vi "Main.vi"() -> ()   [LabVIEW 2015, in "ModbusOverMOXA.lvlib"]
doc: "This template is based from the Queued Message Handler design pattern and the Queued Message Handler Project Template that ships with LabVIEW 2014.\n\nThe main difference is that the Queue is private to this module and communication between modules is done via Broadcast and Requests events.\n\nRequests events are wrapped via public API methods and are handled in the Event handler loop in this VI.\nAny module can register for Broadcast events sent by this module.\n\nThe Event Handling Loop generates messages based on user interface actions.\n\nThe Message Handling Loop processes messages generated by the Event Handling Loop, or by other messages. The messages are string values, so new messages can be added easily to the Message Cases case structure in the Message Handling Loop. Each message cluster can also provide an optional value for Message Data, which is a variant that can be converted to whatever message-specific data is required.\n_____\nBased on Delacor QMH Project Template 3.1.0.34."
uses:
  ModbusOverMOXA.lvlib
  <vilib>/Delacor/Delacor QMH/Libraries/Cloneable Module Admin_class/Delacor_lib_QMH_Cloneable Module Admin.lvclass
  libs/ModBUS.lvlibp/RTU/RTU.lvclass
  Module Data--cluster.ctl
  libs/ModBUS.lvlibp/Base/Modbus.lvclass
  Command.ctl
  <vilib>/Delacor/Delacor QMH/Libraries/Cloneable Module Admin_class/Delacor_lib_QMH_Cloneable Module Admin.lvclass/Delacor_lib_QMH_Cloneable Module Admin.ctl
  Stop Argument--cluster.ctl
  <vilib>/Delacor/Delacor QMH/Libraries/Module Admin_class/Delacor_lib_QMH_Module Admin.lvclass/Delacor_lib_QMH_Module Admin.ctl
  Configure Argument--cluster.ctl
  SetRemote Argument--cluster.ctl
  GetStatus Argument--cluster.ctl
  Drive Argument--cluster.ctl
  ReadRegister Argument--cluster.ctl
  WriteRegister Argument--cluster.ctl
  <vilib>/Utility/miscctls.llb/LVPointTypeDef.ctl
  engage Argument--cluster.ctl
  <vilib>/Delacor/Delacor QMH/Libraries/Cloneable Module Admin_class/Delacor_lib_QMH_Get Module ID.vi
  <vilib>/Delacor/Delacor QMH/Libraries/Module Admin_class/Delacor_lib_QMH_Get External Launch.vi
  <vilib>/Delacor/Delacor QMH/Libraries/Message Queue_class/Delacor_lib_QMH_Enqueue Message (Single).vi
  <vilib>/Utility/error.llb/Error Cluster From Error Code.vi
  <vilib>/ErrorRing/Error Ring.xnode
  <vilib>/Delacor/Delacor QMH/Libraries/Message Queue_class/Delacor_lib_QMH_Message Queue.lvclass
  Clone Registration/Clone Registration.lvlib
  libs/Serializer.lvlibp
  libs/MQTT.lvlibp
panel:
  in  "Simulate MHL Error":bool
  in  "Simulate EHL Error":bool
  out "error out":errorcluster
  in  "Module Admin":refnum<class "Delacor_lib_QMH_Cloneable Module Admin.lvclass">
  out "Status":string
  # "Other QMH Modules communicate with this Module via its Public API (wrappers for its Request Events).\n\nThis Module communicates with other Modules via its Broadcast Events.\nAny module that wants to get these messages, just registers for this module's Broadcast events."
  # "This template is for the Delacor Modified Queued Message Handler design pattern.\n\nSee the block diagram for more information on how to use this template."
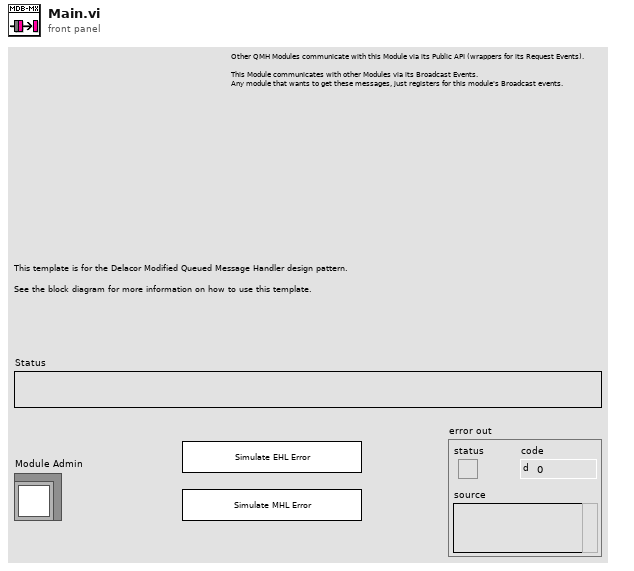
[diagram p1: front panel]
types:
  T1 = typedef "ModbusOverMOXA.lvlib/Request Events--cluster.ctl" = cluster{"Stop Module":refnum<user-event>, "Show Panel":refnum<user-event>, "Hide Panel":refnum<user-event>, "Show Diagram":refnum<user-event>, "Get Module Execution Status":refnum<user-event>, "Configure":refnum<user-event>, "SetRemote":refnum<user-event>, "GetStatus":refnum<user-event>, "engage":refnum<user-event>, "Drive":refnum<user-event>, "ReadRegister":refnum<user-event>, "WriteRegister":refnum<user-event>}
  T2 = typedef "Serializer.lvlibp/Broadcast Events--cluster.ctl" = cluster{"Module Did Init":refnum<user-event>, "Status Updated":refnum<user-event>, "Error Reported":refnum<user-event>, "Module Did Stop":refnum<user-event>, "Update Module Execution Status":refnum<user-event>, "Received":refnum<user-event>}
  T3 = typedef "MQTT.lvlibp/Broadcast Events--cluster.ctl" = cluster{"Module Did Init":refnum<user-event>, "Status Updated":refnum<user-event>, "Error Reported":refnum<user-event>, "Module Did Stop":refnum<user-event>, "Update Module Execution Status":refnum<user-event>, "Message":refnum<user-event>}
  T4 = typedef "ModbusOverMOXA.lvlib/Module Data--cluster.ctl" = cluster{"Status":string, "ModBUS":refnum<class "Modbus.lvclass">, "BitewiseCommand":cluster{"Register":dbl, "Command":string}, "Broadcasts":variant, "Subscriptions":variant, "commands queue":refnum<queue>, "Processing":bool, "processed command":T5, "StatusUpdate":timestamp}
  T5 = typedef "Command.ctl" = cluster{"Command":string, "ByteArray":u8[], "Finished":bool, "Time Stamp":timestamp}
  T6 = typedef "ModbusOverMOXA.lvlib/Stop Argument--cluster.ctl" = cluster{"Origin":string, "Module ID":i32, "Exit via Stop Module Req?":bool, "Wait for Module to stop?":bool}
  T7 = typedef "ModbusOverMOXA.lvlib/Configure Argument--cluster.ctl" = cluster{"Module ID":i32, "Jsonconfig":string}
  T8 = typedef "ModbusOverMOXA.lvlib/SetRemote Argument--cluster.ctl" = cluster{"Module ID":i32, "Remote?":bool}
  T9 = typedef "ModbusOverMOXA.lvlib/GetStatus Argument--cluster.ctl" = cluster{"Module ID":i32, "Boolean":bool}
  T10 = typedef "ModbusOverMOXA.lvlib/Drive Argument--cluster.ctl" = cluster{"Module ID":i32, "Hz":dbl}
  T11 = typedef "ModbusOverMOXA.lvlib/ReadRegister Argument--cluster.ctl" = cluster{"Module ID":i32, "Register":u16, "Length":u16}
  T12 = typedef "ModbusOverMOXA.lvlib/WriteRegister Argument--cluster.ctl" = cluster{"Module ID":i32, "Register":u16, "Data":u16}
  T13 = typedef "LVPointTypeDef.ctl" = cluster{"Horizontal":i16, "Vertical":i16}
  T14 = enum32{"Invalid", "Standard", "Closed", "Hidden", "Minimized", "Maximized"}
  T15 = enum32{"invalid lock state", "Not Locked", "Locked (No Password)", "Password-protected"}
  T16 = typedef "ModbusOverMOXA.lvlib/engage Argument--cluster.ctl" = cluster{"Module ID":i32, "Engage":bool}
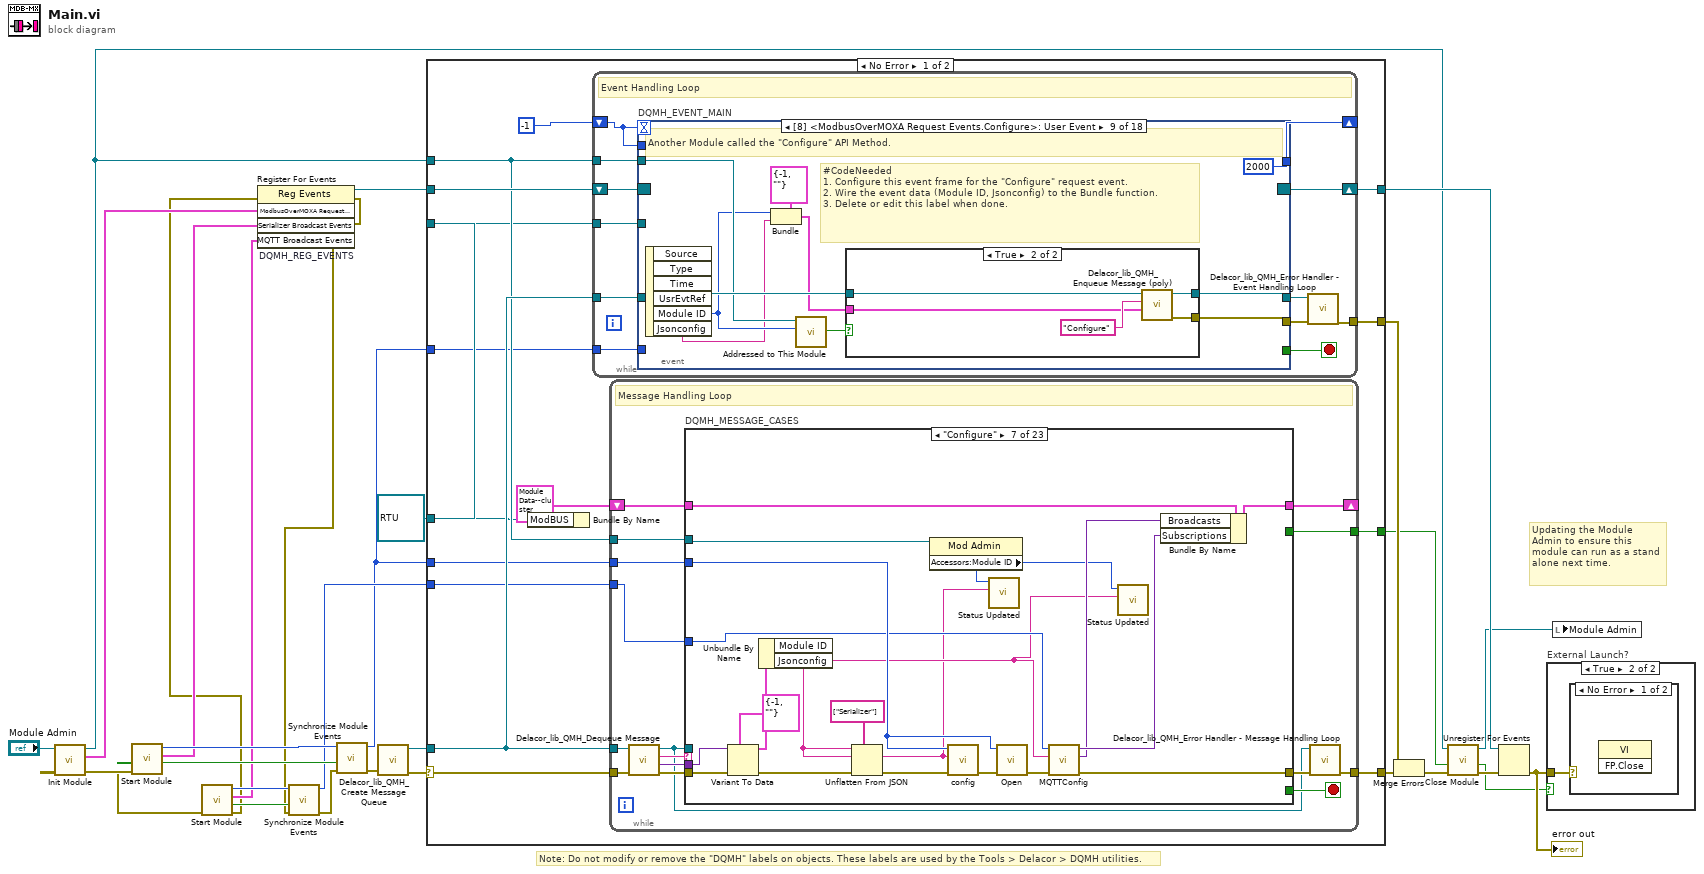
[diagram p0: block diagram]
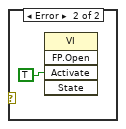
[diagram p3: hidden frame]
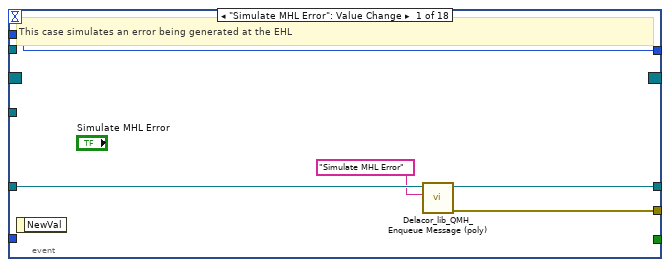
[diagram p4: hidden frame]
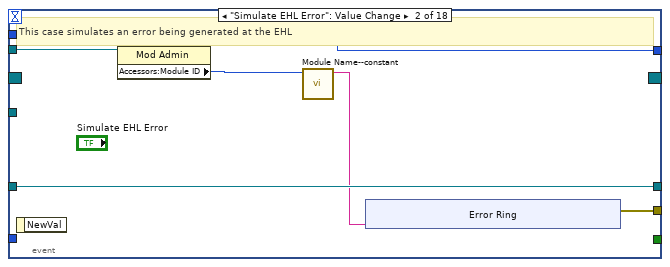
[diagram p5: hidden frame]
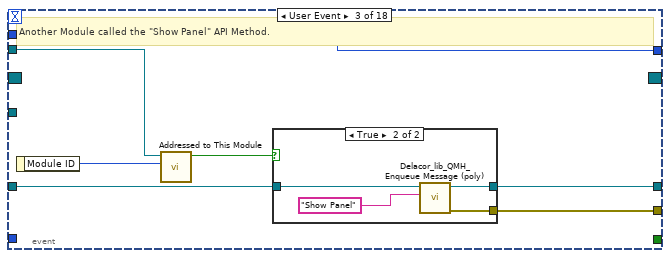
[diagram p6: hidden frame]
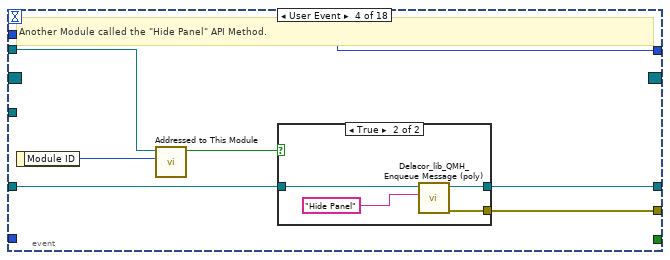
[diagram p8: hidden frame]
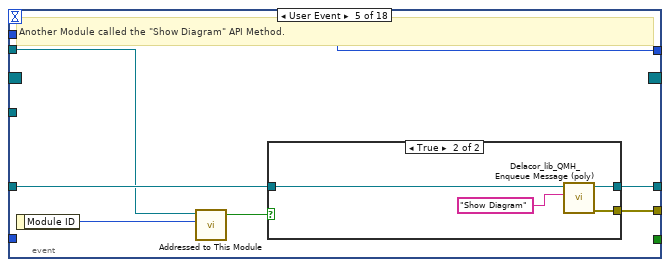
[diagram p10: hidden frame]
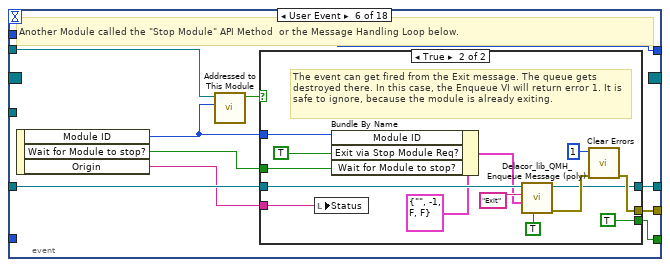
[diagram p12: hidden frame]
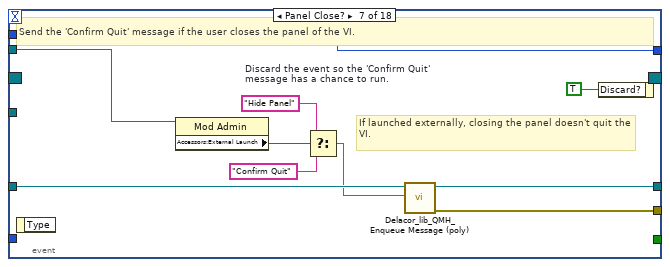
[diagram p14: hidden frame]
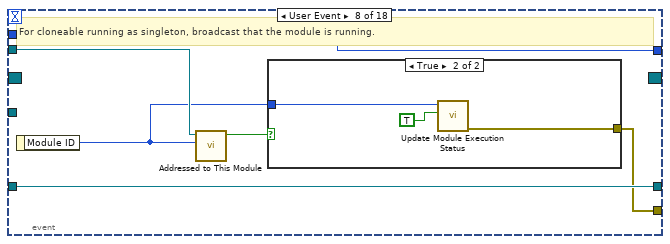
[diagram p15: hidden frame]
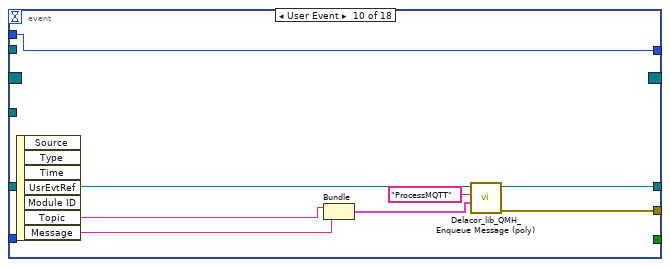
[diagram p18: hidden frame]
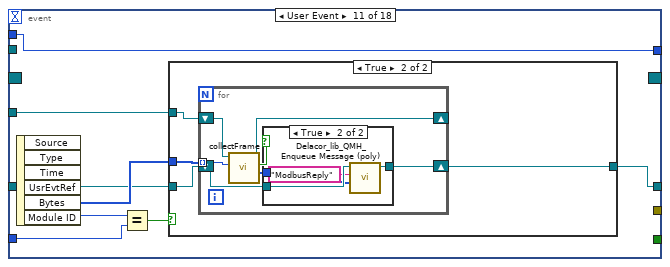
[diagram p19: hidden frame]
diagram:
  w1 = refnum<class "RTU.lvclass"> refnum ("ModBUS.lvlibp:RTU.lvclass")
  # "Note: Do not modify or remove the \"DQMH\" labels on objects. These labels are used by the Tools > Delacor > DQMH utilities."
  # "Updating the Module Admin to ensure this module can run as a stand alone next time."
  n1 = call "Init Module.vi"("Cloneable Module Admin in"="Module Admin") -> ("error out"=w11:errorcluster, "ModbusOverMOXA Request Events"=w25:T1, "Cloneable Module Admin out"=w21:refnum<class "Delacor_lib_QMH_Cloneable Module Admin.lvclass">)  [unwired: 8 in]
  n2 = call "Start Module.vi"("error in (no error)"=w11) -> ("error out"=w4:errorcluster, "Wait for Event Sync?"=w13:bool, "Serializer Broadcast Events"=w12:T2, "Module ID"=w14:i32)  [unwired: 7 in]
  n3 = call "Start Module.vi"("error in (no error)"=w4) -> ("error out"=w3:errorcluster, "Wait for Event Sync?"=w9:bool, "MQTT Broadcast Events"=w8:T3, "Module ID"=w10:i32)  [unwired: 7 in]
  n4 = register-events "DQMH_REG_EVENTS"(error in=w3, w25, w12, w8) -> (reference out=w26:refnum<event-registration>, error out=w6:errorcluster)  [unwired: 1 in]
  n5 = call "Synchronize Module Events.vi"("error in (no error)"=w6, "Wait for Event Sync?"=w9, "Module ID"=w10) -> ("error out"=w5:errorcluster, "Module ID (dup)"=w7:i32)  [unwired: 7 in]
  n6 = call "Synchronize Module Events.vi"("error in (no error)"=w5, "Wait for Event Sync?"=w13, "Module ID"=w14) -> ("error out"=w15:errorcluster, "Module ID (dup)"=w2:i32)  [unwired: 7 in]
  n7 = call <vilib>:"Delacor_lib_QMH_Create Message Queue.vi"("error in (no error)"=w15) -> ("error out"=w16:errorcluster, "Message Queue out"=w24:refnum<class "Delacor_lib_QMH_Message Queue.lvclass">)  [unwired: 9 in]
  n8 = case shown="No Error" w16 {
    selector: w16 -> [w40 w789]
    tunnel: [w46 w789] -> w28
    tunnel: [w45 w790] -> w27
    tunnel: w26 -> [w43 w790]
    tunnel: w24 -> [w42 _]
    tunnel: [w41 _] -> w29
    tunnel: w21 -> [w39 w785]
    tunnel: [w38 _] -> w19
    tunnel: w2 -> [w37 _]
    tunnel: w7 -> [w36 _]
    tunnel: w2 -> [w35 _]
    tunnel: w1 -> [w33 _]
    tunnel: w1 -> [w32 _]
    frame No Error {
      n9 = Bundle By Name(cluster=T4 {"Status"="", "ModBUS"=refnum, "BitewiseCommand"={"Register"=0.0, "Command"=""}, "Broadcasts"=variant, "Subscriptions"=variant, "commands queue"=refnum, "Processing"=FALSE, "processed command"={"Command"="", "ByteArray"=[], "Finished"=FALSE, "Time Stamp"=timestamp(0 s since 1904-01-01)}, "StatusUpdate"=timestamp(0 s since 1904-01-01)} ("Data Cluster"), "ModBUS"=w33) -> (w34:T4)
      n10 = while {
        tunnel: w42 -> [w58]
        shift-right: [w56] -> w45
        shift-left: w43 -> [w57]
        tunnel: [w52] -> w41
        tunnel: w39 -> [w51]
        tunnel: w35 -> [w50]
        tunnel: w32 -> [w49]
        shift-right: [w48] -> _
        shift-left: -1 -> [w47]
        stop <- w54 stop-if-true
        # "Event Handling Loop"
        n11 = event "DQMH_EVENT_MAIN" shown="[8] <ModbusOverMOXA Request Events.Configure>: User Event" {
          selector: w57 -> [_ _ _ _ _ _ _ _ _ _ _ _ _ _ _ _ _ _]
          dyn-events: [_ _ _ _ _ _ _ _ _ _ _ _ _ _ _ _ _ _] -> w56
          timeout: w47 -> [_ _ _ _ _ _ _ _ _ _ _ _ _ _ _ _ _ _]
          tunnel: [_ _ _ _ _ w117 _ _ _ _ _ _ _ _ _ _ _ _] -> w54
          tunnel: w58 -> [w63 w69 w83 w95 w107 w120 w146 w151 w166 w179 w183 w215 w231 w242 w251 w267 w284 w301]
          tunnel: [w61 w68 w81 w93 w103 w122 w145 w150 w160 w177 _ w209 w225 w240 w246 w261 w278 w295] -> w55
          tunnel: [w62 w69 w82 w94 w106 w121 w144 w151 w165 w178 w182 w214 w230 w241 w250 w266 w283 w300] -> w53
          tunnel: w51 -> [_ w67 w78 w90 w104 w119 w140 w152 w163 _ _ w212 w228 _ w248 w264 w281 w298]
          tunnel: w50 -> [_ _ _ _ _ _ _ _ _ _ w187 _ _ _ _ _ _ _]
          tunnel: w49 -> [_ _ _ _ _ _ _ _ _ _ w184 _ _ _ _ _ _ _]
          tunnel: [w59 w64 w77 w89 w101 w113 w138 w148 2000 w180 w181 w206 w222 w238 w243 w258 w274 w291] -> w48
          tunnel: w47 -> [w59 w64 w77 w89 w101 w113 w138 w148 _ w180 w181 w206 w222 w238 w243 w258 w274 w291]
          event "Simulate MHL Error": Value Change {
            # "This case simulates an error being generated at the EHL"
            n12 = event-data() -> ()  [unwired: 1 in, 1 out]
            n13 = call-poly <vilib>:"Delacor_lib_QMH_Enqueue Message (poly).vi"("Message"="Simulate MHL Error", "Message Queue in"=w63) -> ("error out"=w61:errorcluster, "Message Queue out"=w62:refnum<class "Delacor_lib_QMH_Message Queue.lvclass">)  [unwired: 8 in]
          }
          event "Simulate EHL Error": Value Change {
            # "This case simulates an error being generated at the EHL"
            n14 = event-data() -> ()  [unwired: 1 in, 1 out]
            n15 = property class="Mod Admin"(reference=w67) -> ("Accessors:Module ID"=w66:i32)  [unwired: 1 in, 2 out]
            n16 = call "Module Name--constant.vi"("Module ID"=w66) -> ("Module Name"=w65:string)  [unwired: 10 in]
            n17 = xnode "Error Ring"("parameter 0"=w65) -> ("error out"=w68:errorcluster)
          }
          event User Event {
            # "Another Module called the \"Show Panel\" API Method."
            n18 = event-data() -> ("Module ID"=w80:i32)  [unwired: 1 in]
            n19 = call "Addressed to This Module.vi"("Module ID from Argument"=w80, "Module Admin"=w78) -> ("Addressed to this instance?"=w79:bool)  [unwired: 8 in, 1 out]
            n20 = case shown="True" w79 {
              tunnel: w83 -> [w84 w88]
              tunnel: [w84 w87] -> w82
              tunnel: [_ w86] -> w81
              frame False {
              }
              frame True {
                n21 = call-poly <vilib>:"Delacor_lib_QMH_Enqueue Message (poly).vi"("Message"="Show Panel", "Message Queue in"=w88) -> ("error out"=w86:errorcluster, "Message Queue out"=w87:refnum<class "Delacor_lib_QMH_Message Queue.lvclass">)  [unwired: 8 in]
              }
            }
          }
          event User Event {
            # "Another Module called the \"Hide Panel\" API Method."
            n22 = event-data() -> ("Module ID"=w92:i32)  [unwired: 1 in]
            n23 = call "Addressed to This Module.vi"("Module ID from Argument"=w92, "Module Admin"=w90) -> ("Addressed to this instance?"=w91:bool)  [unwired: 8 in, 1 out]
            n24 = case shown="True" w91 {
              tunnel: w95 -> [w96 w100]
              tunnel: [w96 w99] -> w94
              tunnel: [_ w98] -> w93
              frame False {
              }
              frame True {
                n25 = call-poly <vilib>:"Delacor_lib_QMH_Enqueue Message (poly).vi"("Message"="Hide Panel", "Message Queue in"=w100) -> ("error out"=w98:errorcluster, "Message Queue out"=w99:refnum<class "Delacor_lib_QMH_Message Queue.lvclass">)  [unwired: 8 in]
              }
            }
          }
          event User Event {
            # "Another Module called the \"Show Diagram\" API Method."
            n26 = event-data() -> ("Module ID"=w102:i32)  [unwired: 1 in]
            n27 = call "Addressed to This Module.vi"("Module ID from Argument"=w102, "Module Admin"=w104) -> ("Addressed to this instance?"=w105:bool)  [unwired: 8 in, 1 out]
            n28 = case shown="True" w105 {
              tunnel: w107 -> [w108 w112]
              tunnel: [w108 w111] -> w106
              tunnel: [_ w109] -> w103
              frame False {
              }
              frame True {
                n29 = call-poly <vilib>:"Delacor_lib_QMH_Enqueue Message (poly).vi"("Message"="Show Diagram", "Message Queue in"=w112) -> ("error out"=w109:errorcluster, "Message Queue out"=w111:refnum<class "Delacor_lib_QMH_Message Queue.lvclass">)  [unwired: 8 in]
              }
            }
          }
          event User Event {
            # "Another Module called the \"Stop Module\" API Method  or the Message Handling Loop below."
            n30 = event-data() -> ("Module ID"=w115:i32, "Wait for Module to stop?"=w116:bool, "Origin"=w114:string)  [unwired: 1 in]
            n31 = call "Addressed to This Module.vi"("Module ID from Argument"=w115, "Module Admin"=w119) -> ("Addressed to this instance?"=w118:bool)  [unwired: 8 in, 1 out]
            n32 = case shown="True" w118 {
              tunnel: [_ w133] -> w122
              tunnel: [w123 w132] -> w121
              tunnel: w120 -> [w123 w131]
              tunnel: [_ TRUE] -> w117
              tunnel: w116 -> [_ w126]
              tunnel: w115 -> [_ w128]
              tunnel: w114 -> [_ w124]
              frame False {
              }
              frame True {
                # "The event can get fired from the Exit message. The queue gets destroyed there. In this case, the Enqueue VI will return error 1. It is safe to ignore, because the module is already exiting."
                n33 = local write "Status"(w124) -> ()
                n34 = Bundle By Name(cluster=T6 {"Origin"="", "Module ID"=-1, "Exit via Stop Module Req?"=FALSE, "Wait for Module to stop?"=FALSE} ("Stop Argument"), "Module ID"=w128, "Exit via Stop Module Req?"=TRUE, "Wait for Module to stop?"=w126) -> (w125:T6)
                n35 = call-poly <vilib>:"Delacor_lib_QMH_Enqueue Message (poly).vi"("Priority Message? (F)"=TRUE, "Message Data"=w125, "Message"="Exit", "Message Queue in"=w131) -> ("error out"=w136:errorcluster, "Message Queue out"=w132:refnum<class "Delacor_lib_QMH_Message Queue.lvclass">)  [unwired: 6 in]
                n36 = call <vilib>:"Clear Errors.vi"("error in (no error)"=w136, "specific error code to clear (0: all)"=1) -> ("error out"=w133:errorcluster)  [unwired: 4 in, 1 out]
              }
            }
          }
          event Panel Close? {
            w147 = TRUE  # Discard the event so the 'Confirm Quit' message has a chance to run.
            # "If launched externally, closing the panel doesn't quit the VI."
            # "Send the 'Confirm Quit' message if the user closes the panel of the VI."
            n37 = event-data() -> ()  [unwired: 1 in, 1 out]
            n38 = property class="Mod Admin"(reference=w140) -> ("Accessors:External Launch"=w139:bool)  [unwired: 1 in, 2 out]
            n39 = Select(t="Hide Panel" ("Message"), s=w139, f="Confirm Quit" ("Message")) -> (s? t:f=w141:string)
            n40 = call-poly <vilib>:"Delacor_lib_QMH_Enqueue Message (poly).vi"("Message"=w141, "Message Queue in"=w146) -> ("error out"=w145:errorcluster, "Message Queue out"=w144:refnum<class "Delacor_lib_QMH_Message Queue.lvclass">)  [unwired: 8 in]
            n41 = event-data("Discard?"=w147) -> ()  [unwired: 1 in, 1 out]
          }
          event User Event {
            # "For cloneable running as singleton, broadcast that the module is running."
            n42 = event-data() -> ("Module ID"=w149:i32)  [unwired: 1 in]
            n43 = call "Addressed to This Module.vi"("Module ID from Argument"=w149, "Module Admin"=w152) -> ("Addressed to this instance?"=w153:bool)  [unwired: 8 in, 1 out]
            n44 = case shown="True" w153 {
              tunnel: [_ w156] -> w150
              tunnel: w149 -> [_ w155]
              frame False {
              }
              frame True {
                n45 = call "Update Module Execution Status.vi"("Running?"=TRUE, "Module ID"=w155) -> ("error out"=w156:errorcluster)  [unwired: 9 in]
              }
            }
          }
          event User Event {
            # "#CodeNeeded\n1. Configure this event frame for the \"Configure\" request event.\n2. Wire the event data (Module ID, Jsonconfig) to the Bundle function.\n3. Delete or edit this label when done."
            # "Another Module called the \"Configure\" API Method."
            n46 = event-data() -> ("Module ID"=w159:i32, "Jsonconfig"=w158:string)  [unwired: 1 in, 4 out]
            n47 = Bundle(cluster=T7 {"Module ID"=-1, "Jsonconfig"=""} ("Configure Argument"), "Module ID"=w159, "Jsonconfig"=w158) -> (w161:T7)
            n48 = call "Addressed to This Module.vi"("Module ID from Argument"=w159, "Module Admin"=w163) -> ("Addressed to this instance?"=w164:bool)  [unwired: 8 in, 1 out]
            n49 = case shown="True" w164 {
              tunnel: w166 -> [w167 w172]
              tunnel: [w167 w171] -> w165
              tunnel: w161 -> [_ w169]
              tunnel: [_ w168] -> w160
              frame False {
              }
              frame True {
                n50 = call-poly <vilib>:"Delacor_lib_QMH_Enqueue Message (poly).vi"("Message Data"=w169, "Message"="Configure", "Message Queue in"=w172) -> ("error out"=w168:errorcluster, "Message Queue out"=w171:refnum<class "Delacor_lib_QMH_Message Queue.lvclass">)  [unwired: 7 in]
              }
            }
          }
          event User Event {
            n51 = event-data() -> ("Topic"=w175:string, "Message"=w174:string)  [unwired: 1 in, 5 out]
            n52 = Bundle("Topic"=w175, "Message"=w174) -> (w173:cluster{"Topic":string, "Message":string})  [unwired: 1 in]
            n53 = call-poly <vilib>:"Delacor_lib_QMH_Enqueue Message (poly).vi"("Message Data"=w173, "Message"="ProcessMQTT", "Message Queue in"=w179) -> ("error out"=w177:errorcluster, "Message Queue out"=w178:refnum<class "Delacor_lib_QMH_Message Queue.lvclass">)  [unwired: 7 in]
          }
          event User Event {
            n54 = event-data() -> ("Bytes"=w185:u8[], "Module ID"=w188:i32)  [unwired: 1 in, 4 out]
            n55 = Equal?(x=w188, y=w187) -> (x = y?=w186:bool)
            n56 = case shown="True" w186 {
              tunnel: w185 -> [_ w193]
              tunnel: w184 -> [_ w192]
              tunnel: w183 -> [w189 w191]
              tunnel: [w189 w190] -> w182
              frame False {
              }
              frame True {
                n57 = for {
                  tunnel: w193 -> [w199] mode=indexing
                  shift-right: [w197] -> _
                  shift-left: w192 -> [w200]
                  shift-right: [w194] -> w190
                  shift-left: w191 -> [w195]
                  n58 = call-dynamic "collectFrame.vi"("byte"=w199, "RTU in"=w200) -> ("Data"=w196:i16[], "Finished"=w198:bool, "RTU out"=w197:refnum<class "RTU.lvclass">)  [unwired: 5 in, 2 out]
                  n59 = case shown="True" w198 {
                    tunnel: w196 -> [_ w204]
                    tunnel: w195 -> [w201 w205]
                    tunnel: [w201 w202] -> w194
                    frame False {
                    }
                    frame True {
                      n60 = call-poly <vilib>:"Delacor_lib_QMH_Enqueue Message (poly).vi"("Message Data"=w204, "Message"="ModbusReply", "Message Queue in"=w205) -> ("Message Queue out"=w202:refnum<class "Delacor_lib_QMH_Message Queue.lvclass">)  [unwired: 7 in, 1 out]
                    }
                  }
                }
              }
            }
          }
          event User Event {
            # "#CodeNeeded\n1. Configure this event frame for the \"SetRemote\" request event.\n2. Wire the event data (Module ID, Remote?) to the Bundle function.\n3. Delete or edit this label when done."
            # "Another Module called the \"SetRemote\" API Method."
            n61 = event-data() -> ("Module ID"=w208:i32, "Remote?"=w207:bool)  [unwired: 1 in, 4 out]
            n62 = Bundle(cluster=T8 {"Module ID"=-1, "Remote?"=FALSE} ("SetRemote Argument"), "Module ID"=w208, "Remote?"=w207) -> (w210:T8)
            n63 = call "Addressed to This Module.vi"("Module ID from Argument"=w208, "Module Admin"=w212) -> ("Addressed to this instance?"=w213:bool)  [unwired: 8 in, 1 out]
            n64 = case shown="True" w213 {
              tunnel: w215 -> [w216 w221]
              tunnel: [w216 w220] -> w214
              tunnel: w210 -> [_ w218]
              tunnel: [_ w217] -> w209
              frame False {
              }
              frame True {
                n65 = call-poly <vilib>:"Delacor_lib_QMH_Enqueue Message (poly).vi"("Message Data"=w218, "Message"="SetRemote", "Message Queue in"=w221) -> ("error out"=w217:errorcluster, "Message Queue out"=w220:refnum<class "Delacor_lib_QMH_Message Queue.lvclass">)  [unwired: 7 in]
              }
            }
          }
          event User Event {
            # "#CodeNeeded\n1. Configure this event frame for the \"GetStatus\" request event.\n2. Wire the event data (Module ID, Boolean) to the Bundle function.\n3. Delete or edit this label when done."
            # "Another Module called the \"GetStatus\" API Method."
            n66 = event-data() -> ("Module ID"=w223:i32, "Boolean"=w224:bool)  [unwired: 1 in, 4 out]
            n67 = Bundle(cluster=T9 {"Module ID"=-1, "Boolean"=FALSE} ("GetStatus Argument"), "Module ID"=w223, "Boolean"=w224) -> (w226:T9)
            n68 = call "Addressed to This Module.vi"("Module ID from Argument"=w223, "Module Admin"=w228) -> ("Addressed to this instance?"=w229:bool)  [unwired: 8 in, 1 out]
            n69 = case shown="True" w229 {
              tunnel: w231 -> [w232 w237]
              tunnel: [w232 w236] -> w230
              tunnel: w226 -> [_ w234]
              tunnel: [_ w233] -> w225
              frame False {
              }
              frame True {
                n70 = call-poly <vilib>:"Delacor_lib_QMH_Enqueue Message (poly).vi"("Message Data"=w234, "Message"="GetStatus", "Message Queue in"=w237) -> ("error out"=w233:errorcluster, "Message Queue out"=w236:refnum<class "Delacor_lib_QMH_Message Queue.lvclass">)  [unwired: 7 in]
              }
            }
          }
          event Timeout {
            # "Another Module called the \"GetStatus\" API Method."
            n71 = event-data() -> ()  [unwired: 1 in, 3 out]
            n72 = call-poly <vilib>:"Delacor_lib_QMH_Enqueue Message (poly).vi"("Message"="ProcessQuerry", "Message Queue in"=w242) -> ("error out"=w240:errorcluster, "Message Queue out"=w241:refnum<class "Delacor_lib_QMH_Message Queue.lvclass">)  [unwired: 8 in]
          }
          event User Event {
            # "#CodeNeeded\n1. Configure this event frame for the \"engage\" request event.\n2. Wire the event data (Module ID, Engage) to the Bundle function.\n3. Delete or edit this label when done."
            # "Another Module called the \"engage\" API Method."
            n73 = event-data() -> ("Module ID"=w244:i32, "Engage"=w245:bool)  [unwired: 1 in, 4 out]
            n74 = Bundle("Module ID"=w244, "Engage"=w245) -> (w247:cluster{"Module ID":i32, "Engage":bool})  [unwired: 1 in]
            n75 = call "Addressed to This Module.vi"("Module ID from Argument"=w244, "Module Admin"=w248) -> ("Addressed to this instance?"=w249:bool)  [unwired: 8 in, 1 out]
            n76 = case shown="True" w249 {
              tunnel: w251 -> [w252 w257]
              tunnel: [w252 w256] -> w250
              tunnel: w247 -> [_ w254]
              tunnel: [_ w253] -> w246
              frame False {
              }
              frame True {
                n77 = call-poly <vilib>:"Delacor_lib_QMH_Enqueue Message (poly).vi"("Message Data"=w254, "Message"="engage", "Message Queue in"=w257) -> ("error out"=w253:errorcluster, "Message Queue out"=w256:refnum<class "Delacor_lib_QMH_Message Queue.lvclass">)  [unwired: 7 in]
              }
            }
          }
          event User Event {
            # "#CodeNeeded\n1. Configure this event frame for the \"Drive\" request event.\n2. Wire the event data (Module ID, Hz) to the Bundle function.\n3. Delete or edit this label when done."
            # "Another Module called the \"Drive\" API Method."
            n78 = event-data() -> ("Module ID"=w259:i32, "Hz"=w260:dbl)  [unwired: 1 in, 4 out]
            n79 = Bundle(cluster=T10 {"Module ID"=-1, "Hz"=0.0} ("Drive Argument"), "Module ID"=w259, "Hz"=w260) -> (w262:T10)
            n80 = call "Addressed to This Module.vi"("Module ID from Argument"=w259, "Module Admin"=w264) -> ("Addressed to this instance?"=w265:bool)  [unwired: 8 in, 1 out]
            n81 = case shown="True" w265 {
              tunnel: w267 -> [w268 w273]
              tunnel: [w268 w272] -> w266
              tunnel: w262 -> [_ w270]
              tunnel: [_ w269] -> w261
              frame False {
              }
              frame True {
                n82 = call-poly <vilib>:"Delacor_lib_QMH_Enqueue Message (poly).vi"("Message Data"=w270, "Message"="Drive", "Message Queue in"=w273) -> ("error out"=w269:errorcluster, "Message Queue out"=w272:refnum<class "Delacor_lib_QMH_Message Queue.lvclass">)  [unwired: 7 in]
              }
            }
          }
          event User Event {
            # "#CodeNeeded\n1. Configure this event frame for the \"ReadRegister\" request event.\n2. Wire the event data (Module ID, Register, Length) to the Bundle function.\n3. Delete or edit this label when done."
            # "Another Module called the \"ReadRegister\" API Method."
            n83 = event-data() -> ("Module ID"=w275:i32, "Register"=w277:u16, "Length"=w276:u16)  [unwired: 1 in, 4 out]
            n84 = Bundle(cluster=T11 {"Module ID"=-1, "Register"=0, "Length"=1} ("ReadRegister Argument"), "Module ID"=w275, "Register"=w277, "Length"=w276) -> (w279:T11)
            n85 = call "Addressed to This Module.vi"("Module ID from Argument"=w275, "Module Admin"=w281) -> ("Addressed to this instance?"=w282:bool)  [unwired: 8 in, 1 out]
            n86 = case shown="True" w282 {
              tunnel: w284 -> [w285 w290]
              tunnel: [w285 w289] -> w283
              tunnel: w279 -> [_ w287]
              tunnel: [_ w286] -> w278
              frame False {
              }
              frame True {
                n87 = call-poly <vilib>:"Delacor_lib_QMH_Enqueue Message (poly).vi"("Message Data"=w287, "Message"="ReadRegister", "Message Queue in"=w290) -> ("error out"=w286:errorcluster, "Message Queue out"=w289:refnum<class "Delacor_lib_QMH_Message Queue.lvclass">)  [unwired: 7 in]
              }
            }
          }
          event User Event {
            # "#CodeNeeded\n1. Configure this event frame for the \"WriteRegister\" request event.\n2. Wire the event data (Module ID, Register, Data) to the Bundle function.\n3. Delete or edit this label when done."
            # "Another Module called the \"WriteRegister\" API Method."
            n88 = event-data() -> ("Module ID"=w292:i32, "Register"=w294:u16, "Data"=w293:u16)  [unwired: 1 in, 4 out]
            n89 = Bundle(cluster=T12 {"Module ID"=-1, "Register"=0, "Data"=0} ("WriteRegister Argument"), "Module ID"=w292, "Register"=w294, "Data"=w293) -> (w296:T12)
            n90 = call "Addressed to This Module.vi"("Module ID from Argument"=w292, "Module Admin"=w298) -> ("Addressed to this instance?"=w299:bool)  [unwired: 8 in, 1 out]
            n91 = case shown="True" w299 {
              tunnel: w301 -> [w302 w307]
              tunnel: [w302 w306] -> w300
              tunnel: w296 -> [_ w304]
              tunnel: [_ w303] -> w295
              frame False {
              }
              frame True {
                n92 = call-poly <vilib>:"Delacor_lib_QMH_Enqueue Message (poly).vi"("Message Data"=w304, "Message"="WriteRegister", "Message Queue in"=w307) -> ("error out"=w303:errorcluster, "Message Queue out"=w306:refnum<class "Delacor_lib_QMH_Message Queue.lvclass">)  [unwired: 7 in]
              }
            }
          }
        }
        n93 = call-dynamic "Delacor_lib_QMH_Error Handler - Event Handling Loop.vi"("error in (no error)"=w55, "Message Queue in"=w53) -> ("dup error in"=w52:errorcluster)  [unwired: 8 in, 1 out]
      }
      n94 = while {
        tunnel: w42 -> [w314]
        shift-right: [w320] -> _
        shift-left: w34 -> [w321]
        tunnel: w40 -> [w318]
        tunnel: [w312] -> w46
        tunnel: w39 -> [w311]
        tunnel: [w310] -> w38
        tunnel: w37 -> [w309]
        tunnel: w36 -> [w308]
        stop <- w319 stop-if-true
        # "Message Handling Loop"
        n95 = call-dynamic "Delacor_lib_QMH_Dequeue Message.vi"("error in (no error)"=w318, "Message Queue in"=w314) -> ("error out"=w317:errorcluster, "Message Data"=w315:variant, "Message"=w316:string, "Message Queue out"=w313:refnum<class "Delacor_lib_QMH_Message Queue.lvclass">)  [unwired: 6 in]
        n96 = case "DQMH_MESSAGE_CASES" shown="\"Configure\"" w316 {
          selector: w316 -> [_ _ _ _ _ _ _ _ _ _ w465 w485 w508 _ _ _ _ _ _ _ _ _ w772]
          tunnel: w313 -> [_ _ _ _ _ _ _ _ w418 w438 w458 w478 w501 _ w528 w592 w632 _ w707 _ w740 w766 _]
          tunnel: w317 -> [w337 w353 w361 w367 w370 w391 w411 w417 w435 w457 w477 w500 w523 w526 w533 w601 w646 w705 w716 w729 w739 w768 _]
          tunnel: [w330 w354 w361 w367 w369 w389 w396 w415 w420 w439 w459 w479 w502 w524 w534 w602 w649 w703 w706 w727 w738 w763 w773] -> w322
          tunnel: w321 -> [w336 w355 w360 w366 w371 w390 w410 w416 w437 w448 w473 w496 w519 w525 w532 w597 w648 w704 w715 w728 w743 w746 w774]
          tunnel: [w335 w355 w360 w366 w371 w390 w399 w416 w437 w448 w473 w496 w519 w525 w531 w597 w647 w704 w715 w728 w743 w746 w774] -> w320
          tunnel: [_ _ _ _ _ _ _ _ _ _ _ _ _ _ _ _ _ _ _ _ _ w765 _] -> w319
          tunnel: w315 -> [_ w352 _ _ _ _ w409 w414 _ w456 w476 w499 w522 _ _ w600 w644 _ w714 _ _ w759 _]
          tunnel: w311 -> [w327 w347 w358 w365 w368 _ w395 _ _ _ _ _ _ _ w527 w588 w640 _ w711 w724 _ w755 w770]
          tunnel: [_ _ _ _ _ _ _ _ _ _ _ _ _ _ _ _ _ _ _ _ _ w757 _] -> w310
          tunnel: w309 -> [_ _ _ _ _ _ w402 _ _ _ _ _ _ _ w529 _ _ _ _ _ _ w751 _]
          tunnel: w308 -> [_ _ _ _ _ _ w400 _ _ _ _ _ _ _ _ _ w637 _ _ _ _ w749 _]
          frame "Initialize" {
            w334 = "Initial Message" ("Initial Message")
            # "Initialize - Any operation that needs to be done before the module can receive messages. Synchronize Caller Events.vi will inform Start Module.vi that the module has launched and is ready to receive messages. Module Did Init.vi will broadcast that the module initialized."
            n97 = call "Synchronize Caller Events.vi"("error in (no error)"=w337, "Module Admin"=w327) -> ("error out"=w331:errorcluster, "Module Admin out"=w326:refnum<class "Delacor_lib_QMH_Cloneable Module Admin.lvclass">)  [unwired: 8 in]
            n98 = property class="Mod Admin"(reference=w326) -> ("Accessors:Module ID"=w329:i32, "Accessors:External Launch"=w328:bool)  [unwired: 1 in, 2 out]
            n99 = call "Module Name--constant.vi"("Module ID"=w329) -> ("Module Name"=w341:string)  [unwired: 10 in]
            n100 = Obtain Queue(element data type=T5 {"Command"="", "ByteArray"=[], "Finished"=FALSE, "Time Stamp"=timestamp(0 s since 1904-01-01)} ("Cluster")) -> (queue out=w323:refnum<queue>)  [unwired: 4 in, 2 out]
            n101 = property class="VI"("Front Panel.Title"=w341) -> (reference out=w344:refnum<vi>, error out=w345:errorcluster)  [unwired: 2 in]
            n102 = Select(t=T14."Hidden" ("State"), s=w328, f=T14."Standard" ("State")) -> (s? t:f=w338:T14)
            n103 = Bundle By Name(cluster=w336, "commands queue"=w323, "Status"=w334) -> (w335:T4)
            n104 = invoke class="VI" method="FP.Open"(reference=w344, error in=w345, "State"=w338) -> (reference out=w343:refnum<vi>, error out=w342:errorcluster)  [unwired: 2 in, 3 out]
            n105 = call "Module Name--constant.vi"("Module ID"=w329) -> ("Module Name"=w332:string)  [unwired: 10 in]
            n106 = local write "Status"(w334) -> ()
            n107 = invoke class="VI" method="FP.Center"(reference=w343, error in=w342) -> ()  [unwired: 1 in, 3 out]
            n108 = property on="Pane" class="Pane"("Origin"=T13 {"Horizontal"=0, "Vertical"=0}) -> ()  [unwired: 2 in, 2 out]
            n109 = call "Module Did Init.vi"("error in (no error)"=w331, "Initialized?"=TRUE, "Origin"=w332, "Module ID"=w329) -> ("error out"=w330:errorcluster)  [unwired: 7 in]
          }
          frame "Update Display" {
            # "Broadcast updated status to any VI registered to listen to this module's broadcast events."
            # "Convert the message data to a string to display in the Status indicator."
            # "#CodeRecommended - If you wish to decouple the Message Handling Loop from your user interface, consider creating User Events (like the \"Stop\" event in this VI) to message the Event Handling Loop whenever the user interface needs updating."
            # "Update Display - Update user interface here."
            n110 = Variant To Data(error in=w353, type="", Variant=w352) -> (data=w350:string, error out=w349:errorcluster)
            "Status" <- w350
            n111 = property class="Mod Admin"(reference=w347) -> ("Accessors:Module ID"=w346:i32)  [unwired: 1 in, 2 out]
            n112 = call "Status Updated.vi"("error in (no error)"=w349, "Status"=w350, "Module ID"=w346) -> ("error out"=w348:errorcluster)  [unwired: 8 in]
            n113 = Merge Errors(w348) -> (w354:errorcluster)
          }
          frame "Show Panel" {
            # "Show the panel of this VI, and send a status updated message to let listeners know."
            n114 = property class="Mod Admin"(reference=w358) -> ("Accessors:Module ID"=w357:i32)  [unwired: 1 in, 2 out]
            n115 = call "Status Updated.vi"("Status"="Panel shown." ("format string"), "Module ID"=w357) -> ()  [unwired: 9 in, 1 out]
            n116 = invoke class="VI" method="FP.Open"("Activate"=TRUE ("Activate?")) -> ()  [unwired: 4 in, 5 out]
          }
          frame "Hide Panel" {
            # "Hide the panel of this VI, and send a status updated message to let listeners know."
            n117 = property class="Mod Admin"(reference=w365) -> ("Accessors:Module ID"=w364:i32)  [unwired: 1 in, 2 out]
            n118 = call "Status Updated.vi"("Status"="Panel hidden." ("format string"), "Module ID"=w364) -> ()  [unwired: 9 in, 1 out]
            n119 = invoke class="VI" method="FP.Open"("State"=T14."Hidden") -> ()  [unwired: 4 in, 5 out]
          }
          frame "Show Diagram" {
            # "Show Diagram - Show the block diagram of this VI. Used as a debugging tool. There is a button in the module tester that fires the Show Diagram request, which runs this message. Note that the diagram will not be displayed if it is password-protected and the password is not in the cache."
            n120 = disable-structure shown="RUN_TIME_ENGINE==False" {
              disable-tunnel: [w380 w388] -> w369
              disable-tunnel: w370 -> [w379 w388]
              disable-tunnel: w368 -> [w372 _]
              frame condition #0 (active) {
                # "functionality not available in exe"
                n121 = invoke class="VI" method="Lock State.Get"(error in=w379) -> (error out=w378:errorcluster, "Get Lock State"=w377:T15, "pwd in cache"=w374:bool)  [unwired: 3 in, 1 out]
                n122 = Equal?(x=T15."Password-protected", y=w377) -> (x = y?=w375:bool)
                n123 = Compound Arithmetic op=AND(w375, invert w374) -> (w373:bool)
                n124 = case shown="False" w373 {
                  tunnel: [w385 w387] -> w380
                  tunnel: w378 -> [w384 w387]
                  tunnel: w372 -> [w381 _]
                  frame False {
                    n125 = property class="Mod Admin"(reference=w381) -> ("Accessors:Module ID"=w382:i32)  [unwired: 1 in, 2 out]
                    n126 = property class="VI"(error in=w384, "BDWin.Open"=TRUE ("Block Diagram Window:Open")) -> (error out=w385:errorcluster)  [unwired: 1 in, 1 out]
                    n127 = call "Status Updated.vi"("Status"="Block Diagram shown." ("format string"), "Module ID"=w382) -> ()  [unwired: 9 in, 1 out]
                  }
                  frame True {
                    # "Password-protected VI, and the password is not in the cache. Do not show the diagram."
                  }
                }
              }
              frame condition #1 {
              }
            }
          }
          frame "--- Module Specific ---" {
            # "Separator -- The following cases handle messages specific to this Module."
            n128 = Merge Errors(w391) -> (w389:errorcluster)
          }
          frame "Configure" {
            n129 = Variant To Data(error in=w411, type=T7 {"Module ID"=-1, "Jsonconfig"=""} ("Configure Argument"), Variant=w409) -> (data=w407:T7, error out=w406:errorcluster)
            n130 = Unbundle By Name(w407) -> ("Jsonconfig"=w393:string)  [unwired: 1 out]
            n131 = Unflatten From JSON(path=string[] ["Serializer"], JSON string=w393, type and defaults=w393, error in (no error)=w406) -> (value=w392:string, error out=w404:errorcluster)  [unwired: 3 in]
            n132 = property class="Mod Admin"(reference=w395) -> ("Accessors:Module ID"=w394:i32)  [unwired: 1 in, 2 out]
            n133 = call "config.vi"("error in (no error)"=w404, "config"=w392, "Module ID"=w402) -> ("error out"=w403:errorcluster)  [unwired: 8 in]
            n134 = call "Status Updated.vi"("Status"=w392, "Module ID"=w394) -> ()  [unwired: 9 in, 1 out]
            n135 = call "Open.vi"("error in (no error)"=w403, "Module ID"=w402) -> ("error out"=w401:errorcluster)  [unwired: 9 in]
            n136 = call "MQTTConfig.vi"("error in (no error)"=w401, "Jsonconfig"=w393, "Module ID"=w400) -> ("error out"=w396:errorcluster, "Broadcasts"=w397:variant, "Subscriptions"=w398:variant)  [unwired: 6 in]
            n137 = call "Status Updated.vi"("Status"=w393, "Module ID"=w394) -> ()  [unwired: 9 in, 1 out]
            n138 = Bundle By Name(cluster=w410, "Broadcasts"=w397, "Subscriptions"=w398) -> (w399:T4)
          }
          frame "SetRemote" {
            # "Sets inverter in remote operation mode or in manual(local) operation mode"
            n139 = Variant To Data(error in=w417, type=T8 {"Module ID"=-1, "Remote?"=FALSE} ("SetRemote Argument"), Variant=w414) -> (data=w412:T8, error out=w415:errorcluster)
            n140 = Unbundle By Name(w412) -> ()  [unwired: 2 out]
          }
          frame "GetStatus" {
            n141 = Unbundle By Name(w437) -> ("commands queue"=w424:refnum<queue>, "ModBUS"=w436:refnum<class "Modbus.lvclass">)
            n142 = call-dynamic "collectFrame.vi"("Reset"=TRUE, "error in (no error)"=w435, "byte"=u8 0, "Modbus in"=w436) -> ("error out"=w431:errorcluster, "Modbus out"=w432:refnum<class "Modbus.lvclass">)  [unwired: 3 in, 3 out]
            n143 = call-dynamic "0x03ReadHoldingRegisters.vi"("Length 2"=u16 6, "error in (no error)"=w431, "Register"=u16 8, "Addressc"=u8 1, "Modbus in"=w432) -> ("error out"=w422:errorcluster, "Frame"=w427:string)  [unwired: 4 in, 1 out]
            n144 = String To Byte Array(string=w427) -> (unsigned byte array=w426:u8[])
            n145 = call "BuildCommand.vi"("unsigned byte array"=w426, "String"="GetStatus") -> ("command"=w423:T5)  [unwired: 9 in]
            n146 = Enqueue Element(queue=w424, element=w423, error in (no error)=w422) -> (error out=w421:errorcluster)  [unwired: 1 in, 2 out]
            n147 = call-poly <vilib>:"Delacor_lib_QMH_Enqueue Message (poly).vi"("error in (no error)"=w421, "Message"="ProcessQuerry", "Message Queue in"=w418) -> ("error out"=w420:errorcluster)  [unwired: 7 in, 1 out]
          }
          frame "ReadRegister" {
            n148 = Unbundle By Name(w448) -> ("commands queue"=w444:refnum<queue>, "ModBUS"=w447:refnum<class "Modbus.lvclass">)
            n149 = Variant To Data(error in=w457, type=T11 {"Module ID"=-1, "Register"=0, "Length"=1} ("ReadRegister Argument"), Variant=w456) -> (data=w454:T11, error out=w449:errorcluster)
            n150 = Unbundle By Name(w454) -> ("Register"=w451:u16, "Length"=w450:u16)  [unwired: 1 out]
            n151 = call-dynamic "0x03ReadHoldingRegisters.vi"("Length 2"=w450, "error in (no error)"=w449, "Register"=w451, "Addressc"=u8 1, "Modbus in"=w447) -> ("error out"=w442:errorcluster, "Frame"=w453:string)  [unwired: 4 in, 1 out]
            n152 = String To Byte Array(string=w453) -> (unsigned byte array=w445:u8[])
            n153 = call "BuildCommand.vi"("unsigned byte array"=w445, "String"="ReadRegister" ("Frame")) -> ("command"=w443:T5)  [unwired: 9 in]
            n154 = Enqueue Element(queue=w444, element=w443, error in (no error)=w442) -> (error out=w440:errorcluster)  [unwired: 1 in, 2 out]
            n155 = call-poly <vilib>:"Delacor_lib_QMH_Enqueue Message (poly).vi"("error in (no error)"=w440, "Message"="ProcessQuerry", "Message Queue in"=w438) -> ("error out"=w439:errorcluster)  [unwired: 7 in, 1 out]
          }
          frame "WriteRegister" {
            n156 = Unbundle By Name(w473) -> ("commands queue"=w464:refnum<queue>, "ModBUS"=w472:refnum<class "Modbus.lvclass">)
            n157 = Variant To Data(error in=w477, type=T12 {"Module ID"=-1, "Register"=0, "Data"=0} ("WriteRegister Argument"), Variant=w476) -> (data=w475:T12, error out=w474:errorcluster)
            n158 = Unbundle By Name(w475) -> ("Register"=w469:u16, "Data"=w468:u16)  [unwired: 1 out]
            n159 = call-dynamic "0x06PresetSingleRegister.vi"("Data"=w468, "error in (no error)"=w474, "Register"=w469, "Addressc"=u8 1, "Modbus in"=w472) -> ("error out"=w462:errorcluster, "Frame"=w467:string)  [unwired: 4 in, 1 out]
            n160 = String To Byte Array(string=w467) -> (unsigned byte array=w466:u8[])
            n161 = call "BuildCommand.vi"("unsigned byte array"=w466, "String"=w465) -> ("command"=w463:T5)  [unwired: 9 in]
            n162 = Enqueue Element(queue=w464, element=w463, error in (no error)=w462) -> (error out=w460:errorcluster)  [unwired: 1 in, 2 out]
            n163 = call-poly <vilib>:"Delacor_lib_QMH_Enqueue Message (poly).vi"("error in (no error)"=w460, "Message"="ProcessQuerry", "Message Queue in"=w458) -> ("error out"=w459:errorcluster)  [unwired: 7 in, 1 out]
          }
          frame "engage" {
            n164 = Unbundle By Name(w496) -> ("commands queue"=w484:refnum<queue>, "ModBUS"=w495:refnum<class "Modbus.lvclass">)
            n165 = Variant To Data(error in=w500, type=T16 {"Module ID"=-1, "Engage"=FALSE} ("engage Argument"), Variant=w499) -> (data=w498:T16, error out=w497:errorcluster)
            n166 = Unbundle By Name(w498) -> ("Engage"=w490:bool)  [unwired: 1 out]
            n167 = Select(t=u16 5058 ("Register"), s=w490, f=u16 5057 ("Register")) -> (s? t:f=w489:u16)
            n168 = call-dynamic "0x06PresetSingleRegister.vi"("Data"=w489, "error in (no error)"=w497, "Register"=u16 5, "Addressc"=u8 1, "Modbus in"=w495) -> ("error out"=w482:errorcluster, "Frame"=w493:string)  [unwired: 4 in, 1 out]
            n169 = String To Byte Array(string=w493) -> (unsigned byte array=w486:u8[])
            n170 = call "BuildCommand.vi"("unsigned byte array"=w486, "String"=w485) -> ("command"=w483:T5)  [unwired: 9 in]
            n171 = Enqueue Element(queue=w484, element=w483, error in (no error)=w482) -> (error out=w480:errorcluster)  [unwired: 1 in, 2 out]
            n172 = call-poly <vilib>:"Delacor_lib_QMH_Enqueue Message (poly).vi"("error in (no error)"=w480, "Message"="ProcessQuerry", "Message Queue in"=w478) -> ("error out"=w479:errorcluster)  [unwired: 7 in, 1 out]
          }
          frame "Drive" {
            n173 = Unbundle By Name(w519) -> ("commands queue"=w507:refnum<queue>, "ModBUS"=w518:refnum<class "Modbus.lvclass">)
            n174 = Variant To Data(error in=w523, type=T10 {"Module ID"=-1, "Hz"=0.0} ("Drive Argument"), Variant=w522) -> (data=w521:T10, error out=w520:errorcluster)
            n175 = Unbundle By Name(w521) -> ("Hz"=w513:dbl)  [unwired: 1 out]
            n176 = Multiply(x=w513, y=100.0) -> (x*y=w510:dbl)
            n177 = To Unsigned Word Integer(number=w510) -> (unsigned 16bit integer=w511:u16)
            n178 = call-dynamic "0x06PresetSingleRegister.vi"("Data"=w511, "error in (no error)"=w520, "Register"=u16 4, "Addressc"=u8 1, "Modbus in"=w518) -> ("error out"=w505:errorcluster, "Frame"=w516:string)  [unwired: 4 in, 1 out]
            n179 = String To Byte Array(string=w516) -> (unsigned byte array=w509:u8[])
            n180 = call "BuildCommand.vi"("unsigned byte array"=w509, "String"=w508) -> ("command"=w506:T5)  [unwired: 9 in]
            n181 = Enqueue Element(queue=w507, element=w506, error in (no error)=w505) -> (error out=w503:errorcluster)  [unwired: 1 in, 2 out]
            n182 = call-poly <vilib>:"Delacor_lib_QMH_Enqueue Message (poly).vi"("error in (no error)"=w503, "Message"="ProcessQuerry", "Message Queue in"=w501) -> ("error out"=w502:errorcluster)  [unwired: 7 in, 1 out]
          }
          frame "---Copy This Frame---" {
            # "Duplicate this frame when creating new messages.  Change this comment in the duplicated frame to describe this message."
            n183 = Merge Errors(w526) -> (w524:errorcluster)
          }
          frame "ProcessQuerry" {
            n184 = Unbundle By Name(w532) -> ("Processing"=w530:bool)
            n185 = case shown="True" w530 {
              tunnel: [w541 w580] -> w534
              tunnel: w533 -> [w538 w580]
              tunnel: [w543 w573] -> w531
              tunnel: w532 -> [w542 w575]
              tunnel: w529 -> [w536 _]
              tunnel: w528 -> [w535 _]
              tunnel: w527 -> [_ w572]
              frame False {
                n186 = Unbundle By Name(w542) -> ("commands queue"=w545:refnum<queue>)
                n187 = Dequeue Element(queue=w545, timeout in ms (-1)=0, error in (no error)=w538) -> (element=w537:T5, timed out?=w540:bool, error out=w539:errorcluster)  [unwired: 1 out]
                n188 = case shown="False" w540 {
                  tunnel: [w546 w563] -> w543
                  tunnel: w542 -> [w557 w563]
                  tunnel: [w553 w569] -> w541
                  tunnel: w539 -> [w554 w569]
                  tunnel: w537 -> [w555 _]
                  tunnel: w536 -> [w552 _]
                  tunnel: w535 -> [_ w562]
                  frame False {
                    n189 = Unbundle By Name(w555) -> ("ByteArray"=w551:u8[], "Command"=w550:string)
                    n190 = Bundle By Name(cluster=w557, "Processing"=TRUE, "processed command"=w555) -> (w547:T4)
                    n191 = Equal?(x=w550, y="GetStatus") -> (x = y?=w548:bool)
                    n192 = call "Send.vi"("error in (no error)"=w554, "Bytes"=w551, "Module ID"=w552) -> ("error out"=w553:errorcluster)  [unwired: 8 in]
                    n193 = case shown="False" w548 {
                      tunnel: w547 -> [w558 w561]
                      tunnel: [w558 w560] -> w546
                      frame False {
                      }
                      frame True {
                        n194 = Get Date/Time In Seconds() -> (seconds since 1Jan1904=w559:timestamp)
                        n195 = Bundle By Name(cluster=w561, "StatusUpdate"=w559) -> (w560:T4)
                      }
                    }
                  }
                  frame True {
                    n196 = Unbundle By Name(w563) -> ("StatusUpdate"=w567:timestamp)
                    n197 = Get Date/Time In Seconds() -> (seconds since 1Jan1904=w568:timestamp)
                    n198 = Subtract(x=w568, y=w567) -> (x-y=w566:dbl)
                    n199 = Greater Or Equal?(x=w566, y=2.0) -> (x >= y?=w564:bool)
                    n200 = case shown="True" w564 {
                      tunnel: w562 -> [_ w571]
                      frame False {
                      }
                      frame True {
                        n201 = call-poly <vilib>:"Delacor_lib_QMH_Enqueue Message (poly).vi"("Message"="GetStatus", "Message Queue in"=w571) -> ()  [unwired: 8 in, 2 out]
                      }
                    }
                  }
                }
              }
              frame True {
                n202 = Unbundle By Name(w575) -> ("processed command.Time Stamp"=w578:timestamp)
                n203 = Get Date/Time In Seconds() -> (seconds since 1Jan1904=w576:timestamp)
                n204 = Add(x=w578, y=10.0) -> (x+y=w577:timestamp)
                n205 = Less Or Equal?(x=w577, y=w576) -> (x <= y?=w574:bool)
                n206 = case shown="True" w574 {
                  tunnel: w575 -> [w581 w587]
                  tunnel: [w581 w586] -> w573
                  tunnel: w572 -> [_ w584]
                  frame False {
                  }
                  frame True {
                    n207 = property class="Mod Admin"(reference=w584) -> ("Accessors:Module ID"=w583:i32)  [unwired: 1 in, 2 out]
                    n208 = call "Status Updated.vi"("Status"="Querry timeout", "Module ID"=w583) -> ()  [unwired: 9 in, 1 out]
                    n209 = Bundle By Name(cluster=w587, "Processing"=FALSE) -> (w586:T4)
                  }
                }
              }
            }
          }
          frame "ProcessMQTT" {
            # "Duplicate this frame when creating new messages.  Change this comment in the duplicated frame to describe this message."
            n210 = Unbundle By Name(w597) -> ("Subscriptions"=w596:variant)
            n211 = Variant To Data(error in=w601, type=cluster{"Topic":string, "Message":string} {"Topic"="", "Message"=""} ("output cluster"), Variant=w600) -> (data=w598:cluster{"Topic":string, "Message":string}, error out=w595:errorcluster)
            n212 = Unbundle By Name(w598) -> ("Topic"=w589:string, "Message"=w590:string)
            n213 = Get Variant Attribute(Variant=w596, name=w589, default value (empty Variant)=w589, error in=w595) -> (value=w591:string, error out=w594:errorcluster)  [unwired: 2 out]
            n214 = case shown="Default" w591 {
              tunnel: w594 -> [w610 w616 w627]
              tunnel: [w603 w615 w626] -> w593
              tunnel: w592 -> [_ w618 w629]
              tunnel: w590 -> [w607 w614 w625]
              tunnel: w589 -> [w608 _ _]
              tunnel: w588 -> [w605 _ _]
              frame Default {
                n215 = property class="Mod Admin"(reference=w605) -> ("Accessors:Module ID"=w604:i32)  [unwired: 1 in, 2 out]
                n216 = Format Into String(format string="Unrecognized topic:%s  message%s", w608, w607) -> (resulting string=w606:string)  [unwired: 2 in, 1 out]
                n217 = call "Status Updated.vi"("error in (no error)"=w610, "Status"=w606, "Module ID"=w604) -> ("error out"=w603:errorcluster)  [unwired: 8 in]
              }
              frame "Drive" {
                n218 = Unflatten From JSON(JSON string=w614, type and defaults=0.0) -> (value=w612:dbl)  [unwired: 5 in, 1 out]
                n219 = Bundle(cluster=T10 {"Module ID"=-1, "Hz"=0.0} ("Drive Argument"), "Module ID"=0, "Hz"=w612) -> (w617:T10)
                n220 = call-poly <vilib>:"Delacor_lib_QMH_Enqueue Message (poly).vi"("error in (no error)"=w616, "Message Data"=w617, "Message"="Drive", "Message Queue in"=w618) -> ("error out"=w615:errorcluster)  [unwired: 6 in, 1 out]
              }
              frame "Engage" {
                n221 = Unflatten From JSON(JSON string=w625, type and defaults=FALSE) -> (value=w624:bool)  [unwired: 5 in, 1 out]
                n222 = Bundle(cluster=T16 {"Module ID"=-1, "Engage"=FALSE} ("engage Argument"), "Module ID"=0, "Engage"=w624) -> (w628:T16)
                n223 = call-poly <vilib>:"Delacor_lib_QMH_Enqueue Message (poly).vi"("error in (no error)"=w627, "Message Data"=w628, "Message"="engage", "Message Queue in"=w629) -> ("error out"=w626:errorcluster)  [unwired: 6 in, 1 out]
              }
            }
            n224 = Merge Errors(w593) -> (w602:errorcluster)
          }
          frame "ModbusReply" {
            # "Duplicate this frame when creating new messages.  Change this comment in the duplicated frame to describe this message."
            n225 = Unbundle By Name(w648) -> ("processed command.Command"=w636:string, "Broadcasts"=w638:variant)
            n226 = Variant To Data(error in=w646, type=i16[] [] ("Data"), Variant=w644) -> (data=w642:i16[], error out=w645:errorcluster)
            n227 = property class="Mod Admin"(reference=w640) -> ("Accessors:Module ID"=w639:i32)  [unwired: 1 in, 2 out]
            n228 = case shown="\"ReadRegister\"" w636 {
              tunnel: w642 -> [w656 _ _ w678 w685 w697]
              tunnel: [w651 w664 w667 w668 w680 w692] -> w641
              tunnel: w639 -> [w650 w663 w666 w675 w679 w691]
              tunnel: w638 -> [_ _ _ w674 _ _]
              tunnel: w637 -> [_ _ _ w672 _ _]
              frame Default {
                n229 = for {
                  tunnel: w656 -> [w661] mode=indexing
                  shift-right: [w658] -> w654
                  shift-left: "" -> [w660]
                  n230 = Number To Hexadecimal String(1:i16 4 ("width (-)"), 2:w661) -> (0:w659:string)
                  n231 = Concatenate Strings(w660, w659) -> (w658:string)
                }
                n232 = Format Into String(format string="Unknown reply : %s", w654) -> (resulting string=w652:string)  [unwired: 2 in, 1 out]
                n233 = call "Status Updated.vi"("Status"=w652, "Module ID"=w650) -> ("error out"=w651:errorcluster)  [unwired: 9 in]
              }
              frame "Drive" {
                n234 = call "Status Updated.vi"("Status"="Drive Set" ("format string"), "Module ID"=w663) -> ("error out"=w664:errorcluster)  [unwired: 9 in]
              }
              frame "engage" {
                n235 = call "Status Updated.vi"("Status"="Engage set" ("format string"), "Module ID"=w666) -> ("error out"=w667:errorcluster)  [unwired: 9 in]
              }
              frame "GetStatus" {
                w670 = "Status" ("name")
                n236 = call "decodeStatus.vi"("Data"=w678) -> ("String"=w669:string)  [unwired: 9 in, 1 out]
                n237 = Get Variant Attribute(Variant=w674, name=w670, default value (empty Variant)=w670) -> (value=w671:string)  [unwired: 1 in, 3 out]
                n238 = Format Into String(format string="Status : %s", w669) -> (resulting string=w676:string)  [unwired: 2 in, 1 out]
                n239 = call "Status Updated.vi"("Status"=w676, "Module ID"=w675) -> ("error out"=w673:errorcluster)  [unwired: 9 in]
                n240 = call "Publish.vi"("error in (no error)"=w673, "Payload"=w669, "Topic"=w671, "Module ID"=w672) -> ("error out"=w668:errorcluster)  [unwired: 7 in]
              }
              frame "ReadRegister" {
                n241 = for {
                  tunnel: w685 -> [w690] mode=indexing
                  shift-right: [w687] -> w683
                  shift-left: "" -> [w689]
                  n242 = Number To Hexadecimal String(1:i16 4 ("width (-)"), 2:w690) -> (0:w688:string)
                  n243 = Concatenate Strings(w689, w688) -> (w687:string)
                }
                n244 = Format Into String(format string="Register : %s", w683) -> (resulting string=w681:string)  [unwired: 2 in, 1 out]
                n245 = call "Status Updated.vi"("Status"=w681, "Module ID"=w679) -> ("error out"=w680:errorcluster)  [unwired: 9 in]
              }
              frame "WriteRegister" {
                n246 = for {
                  tunnel: w697 -> [w702] mode=indexing
                  shift-right: [w699] -> w695
                  shift-left: "" -> [w701]
                  n247 = Number To Hexadecimal String(1:i16 4 ("width (-)"), 2:w702) -> (0:w700:string)
                  n248 = Concatenate Strings(w701, w700) -> (w699:string)
                }
                n249 = Format Into String(format string="WriteRegister : %s", w695) -> (resulting string=w693:string)  [unwired: 2 in, 1 out]
                n250 = call "Status Updated.vi"("Status"=w693, "Module ID"=w691) -> ("error out"=w692:errorcluster)  [unwired: 9 in]
              }
            }
            n251 = Bundle By Name(cluster=w648, "Processing"=FALSE, "processed command"=T5 {"Command"="", "ByteArray"=[], "Finished"=FALSE, "Time Stamp"=timestamp(0 s since 1904-01-01)} ("Cluster")) -> (w647:T4)
            n252 = call-poly <vilib>:"Delacor_lib_QMH_Enqueue Message (poly).vi"("Message"="ProcessQuerry", "Message Queue in"=w632) -> ("error out"=w633:errorcluster)  [unwired: 8 in, 1 out]
            n253 = Merge Errors(w633, w641, w645) -> (w649:errorcluster)
          }
          frame "--- Exit and Error Handling---" {
            # "Separator - the following cases handle errors and exit messages."
            n254 = Merge Errors(w705) -> (w703:errorcluster)
          }
          frame "Error" {
            # "#CodeRecommended - If you ever change the name of this \"Error\" message, you'll need to update the name in the Check Loop Error.vi as well."
            # "#CodeRecommended - If the module is running in standalone mode (External Launch = FALSE), this code will pop up an error dialog and call the 'Exit' message if an error occurs. Add more fine-grained error handling here."
            # "Error - Check the error message data and respond accordingly. This message is sent by the \"Error Handler\" VIs at the end of each loop in this application."
            n255 = property class="Mod Admin"(reference=w711) -> ("Accessors:External Launch"=w708:bool, "Accessors:Module ID"=w710:i32)  [unwired: 1 in, 2 out]
            n256 = Variant To Data(error in=w716, type=errorcluster {"status"=FALSE, "code"=0, "source"=""} ("error constant"), Variant=w714) -> (data=w717:errorcluster, error out=w712:errorcluster)
            n257 = call "Error Reported.vi"("Error"=w717, "Module ID"=w710) -> ()  [unwired: 9 in, 1 out]
            n258 = case shown="False" w708 {
              tunnel: [w722 _] -> w709
              tunnel: w707 -> [w721 _]
              tunnel: w717 -> [w718 _]
              frame False {
                # "If the module is running standalone, then pop up an error dialog and call the \"Exit\" message."
                n259 = call <vilib>:"Simple Error Handler.vi"("error in (no error)"=w718) -> ()  [unwired: 4 in, 5 out]
                n260 = call-poly <vilib>:"Delacor_lib_QMH_Enqueue Message (poly).vi"("Priority Message? (F)"=TRUE, "Message"="Exit", "Message Queue in"=w721) -> ("error out"=w722:errorcluster)  [unwired: 7 in, 1 out]
              }
              frame True {
                # "If the module was launched externally, calling the Error Reported broadcast VI is the only action performed by the \"Error\" message. The module's caller can then process the error appropriately."
              }
            }
            n261 = Merge Errors(w712, w709) -> (w706:errorcluster)
            n262 = local write "error out"(w706) -> ()
          }
          frame "Simulate MHL Error" {
            # "Simulate an error occurring at the MHL"
            n263 = property class="Mod Admin"(reference=w724) -> ("Accessors:Module ID"=w725:i32)  [unwired: 1 in, 2 out]
            n264 = call "Module Name--constant.vi"("Module ID"=w725) -> ("Module Name"=w723:string)  [unwired: 10 in]
            n265 = xnode "Error Ring"("parameter 0"=w723) -> ("error out"=w726:errorcluster)
            n266 = Merge Errors(w729, w726) -> (w727:errorcluster)
          }
          frame "Confirm Quit" {
            # "#CodeNeeded - If you want to provide an \"Are you sure\" dialog (or some other notification) before the application exits, place that code here. This message is typically sent from a Panel Close? event."
            # "Confirm Quit - Message that can confirm whether or not the user wants to exit this instance."
            n267 = call-poly <vilib>:"Delacor_lib_QMH_Enqueue Message (poly).vi"("Priority Message? (F)"=TRUE, "error in (no error)"=w739, "Message"="Exit", "Message Queue in"=w740) -> ("error out"=w742:errorcluster)  [unwired: 6 in, 1 out]
            n268 = Merge Errors(w742) -> (w738:errorcluster)
          }
          frame "Exit" {
            w750 = "programStop" ("Origin")
            w761 = 91  # 91: not all Exit messages will have an argument
            w765 = TRUE  # Stop the VI
            # "Release the message queue reference"
            # "Exit - Exit the application."
            n269 = Variant To Data(error in=w768, type=T6 {"Origin"="", "Module ID"=-1, "Exit via Stop Module Req?"=FALSE, "Wait for Module to stop?"=FALSE} ("Stop Argument"), Variant=w759) -> (data=w756:T6, error out=w760:errorcluster)
            n270 = Unbundle By Name(w746) -> ("commands queue"=w745:refnum<queue>)
            n271 = call <vilib>:"Clear Errors.vi"("error in (no error)"=w760, "specific error code to clear (0: all)"=w761) -> ("error out"=w767:errorcluster)  [unwired: 4 in, 1 out]
            n272 = Release Queue(queue=w745, force destroy? (F)=TRUE) -> ()  [unwired: 1 in, 3 out]
            n273 = control-ref of="This VI"() -> (w754:refnum<vi>)
            n274 = call-dynamic "Delacor_lib_QMH_Release Message Queue.vi"("error in (no error)"=w767, "Message Queue"=w766) -> ("error out"=w764:errorcluster)  [unwired: 9 in]
            n275 = call "disconnect.vi"("Module ID"=w749) -> ("error out"=w748:errorcluster)  [unwired: 10 in]
            n276 = call "Handle Exit.vi"("Stop Argument"=w756, "Module Admin in"=w755, "VI reference"=w754) -> ("error out"=w762:errorcluster, "Wait for Stop?"=w757:bool)  [unwired: 7 in]
            n277 = call "close.vi"("Module ID"=w751) -> ("error out"=w753:errorcluster)  [unwired: 10 in]
            n278 = call "Stop Module.vi"("error in (no error)"=w748, "Origin"=w750, "Module ID"=w749) -> ("error out"=w747:errorcluster)  [unwired: 8 in]
            n279 = call "Stop Module.vi"("error in (no error)"=w753, "Origin"=w750, "Module ID"=w751) -> ("error out"=w752:errorcluster)  [unwired: 8 in]
            n280 = Merge Errors(w747, w752, w762, w764) -> (w763:errorcluster)
          }
          frame Default {
            # "'Default' case only runs if there is a message that isn't defined in any of the other cases.  Output a programming error."
            n281 = property class="Mod Admin"(reference=w770) -> ("Accessors:Module ID"=w769:i32)  [unwired: 1 in, 2 out]
            n282 = call "Module Name--constant.vi"("Module ID"=w769) -> ("Module Name"=w771:string)  [unwired: 10 in]
            n283 = xnode "Error Ring"("parameter 0"=w772, "parameter 1"=w771) -> ("error out"=w773:errorcluster)
          }
        }
        n284 = call-dynamic "Delacor_lib_QMH_Error Handler - Message Handling Loop.vi"("error in (no error)"=w322, "Message Queue in"=w313) -> ("dup error in"=w312:errorcluster)  [unwired: 8 in, 1 out]
      }
    }
    frame Error {
      n285 = call "Synchronize Caller Events.vi"("Module Admin"=w785) -> ("Module Admin out"=w784:refnum<class "Delacor_lib_QMH_Cloneable Module Admin.lvclass">)  [unwired: 9 in, 1 out]
      n286 = property class="Mod Admin"(reference=w784) -> ("Accessors:Module ID"=w783:i32)  [unwired: 1 in, 2 out]
      n287 = call "Module Name--constant.vi"("Module ID"=w783) -> ("Module Name"=w788:string)  [unwired: 10 in]
      n288 = call "Remove.vi"("Module ID"=w783) -> ()  [unwired: 9 in, 2 out]
      n289 = Format Into String(format string="An error occurred during initialization. %s is no longer running.", w788) -> (resulting string=w786:string)  [unwired: 2 in, 1 out]
      n290 = call "Error Reported.vi"("Additional Information"=w786, "Error"=w789, "Module ID"=w783) -> ()  [unwired: 8 in, 1 out]
    }
  }
  n291 = Merge Errors(w29, w28) -> (w30:errorcluster)
  n292 = call "Close Module.vi"("error in (no error)"=w30, "Wait for stop?"=w19, "Module Admin in"=w21) -> ("error out"=w23:errorcluster, "External Launch"=w17:bool, "Module Admin out"=w20:refnum<class "Delacor_lib_QMH_Cloneable Module Admin.lvclass">)  [unwired: 6 in]
  n293 = Unregister For Events(event registration refnum=w27, error in=w23) -> (error out=w18:errorcluster)
  "error out" <- w18
  n294 = case "External Launch?" shown="True" w17 {
    tunnel: w18 -> [_ w791]
    frame False {
    }
    frame True {
      n295 = case shown="No Error" w791 {
        frame No Error {
          n296 = invoke class="VI" method="FP.Close"() -> ()  [unwired: 3 in, 3 out]
        }
        frame Error {
          n297 = invoke class="VI" method="FP.Open"("Activate"=TRUE ("Activate?")) -> ()  [unwired: 4 in, 5 out]
        }
      }
    }
  }
  n298 = local write "Module Admin"(w20) -> ()
